vi "TraverseControl_High.vi"(0 "Mode":T2=enum."Read traverse position", 1 "Route Checking?":bool, 2 "Home":T1, 3 "Traverse Name":string, 7 "Model       Roll      Pitch       Yaw (deg)":dbl[](array[numeric]) format="%#.2f", 11 "Position input XYZ":dbl[](array[numeric])=[0.0, 0.0, 0.0] format="%.2f", 12 "Last Part of Move?":bool, 13 "Speed Factor":dbl=1.0 min=0.1 max=5.0 format="%.2f", 14 "Backlash Compensation?":bool=TRUE) -> (4 "Position Output XYZ":dbl[](array[numeric]) format="%.2f", 15 "Error String":string)   [LabVIEW 2014]
uses:
  Anemometry/Anemometry Sub Vis/Gen Trav/Trav_mode.ctl
  Anemometry/Anemometry Sub Vis/Controls/Home.ctl
  Anemometry/Anemometry Sub Vis/Globals/Trav_pos_global.vi
  Anemometry/Anemometry Sub Vis/Gen Trav/Route mapping/Route_mapping_global.vi
  Anemometry/Anemometry Sub Vis/Globals/Preference_global.vi
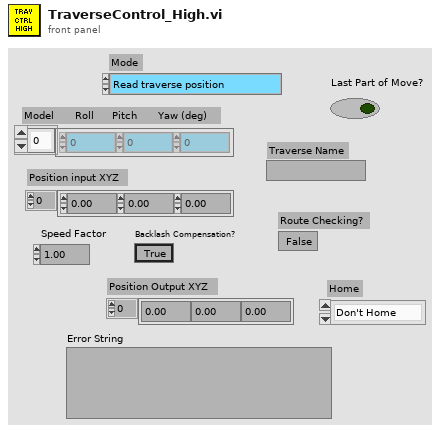
[diagram p1: front panel]
types:
  T1 = typedef "Home.ctl" = enum16{"Don't Home", "Home  +X", "Home  -X", "Home  +Y", "Home  -Y", "Home  +Z", "Home  -Z"}
  T2 = typedef "Trav_mode.ctl" = enum16{"Move traverse", "Read traverse position", "Teach Position"}
  T3 = typedef "Tunnel_Coordinates.ctl" = enum16{"Work in Tunnel Coordinates", "Work in Model Coordinates"}
  T4 = typedef "Box_size.ctl" = cluster{"Max":dbl, "Min":dbl}[]
  T5 = typedef "Exclude_cluster.ctl" = cluster{"Sizes":T4, "Name":string, "Exclude Type":T6}
  T6 = typedef "Exclusion_type.ctl" = enum16{"Exclude completely", "Allow only vertical moves"}
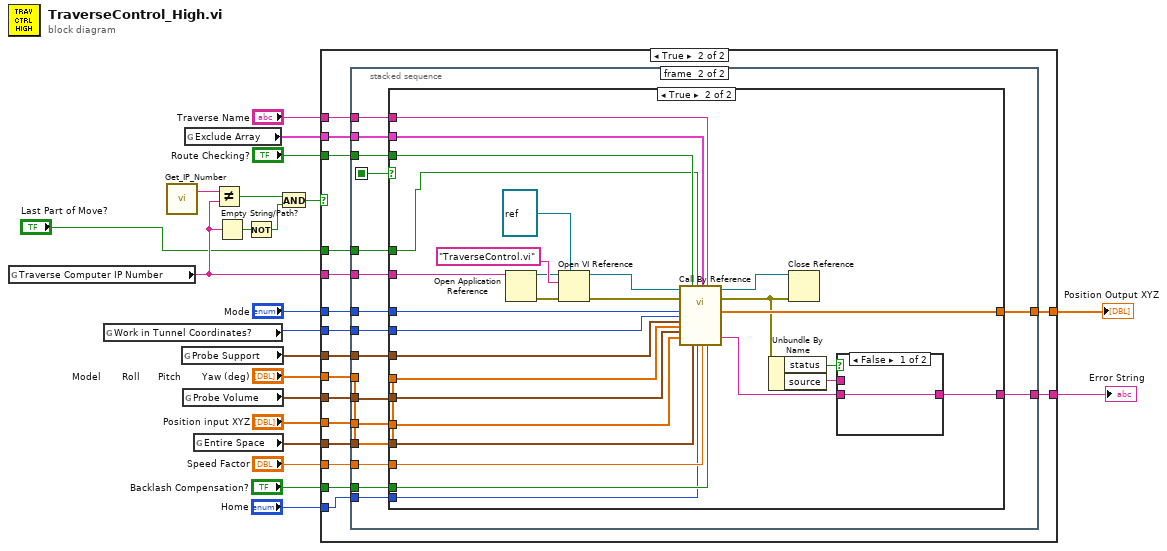
[diagram p0: block diagram]
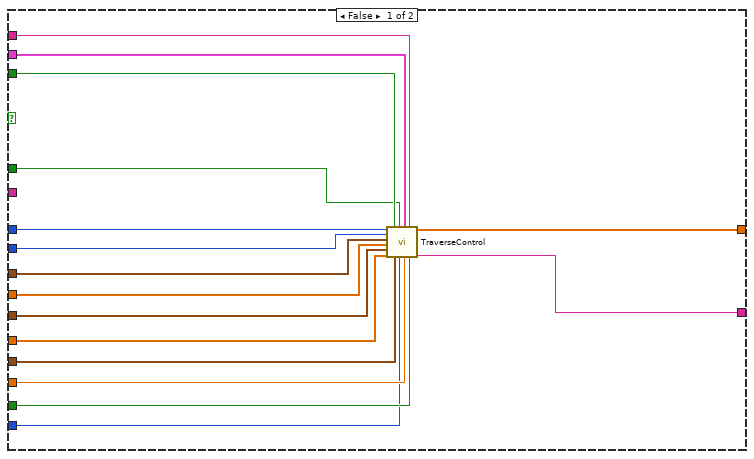
[diagram p2: hidden frame]
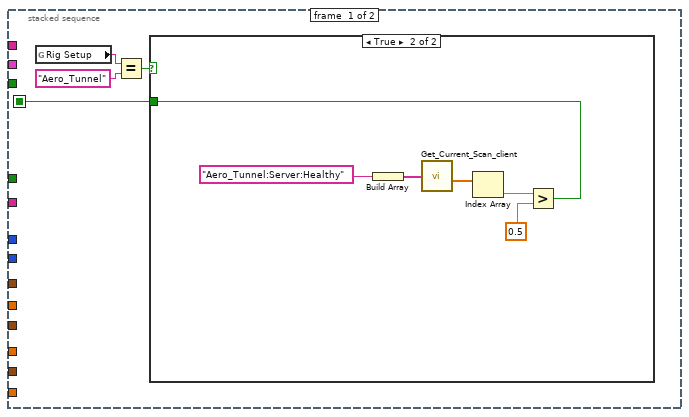
[diagram p3: hidden frame]
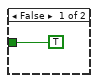
[diagram p4: hidden frame]
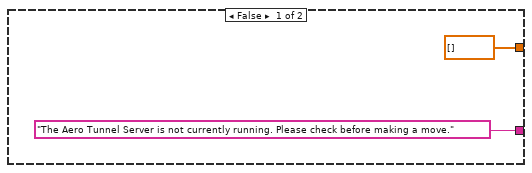
[diagram p5: hidden frame]
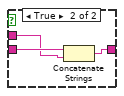
[diagram p6: hidden frame]
diagram:
  n1 = global read "Trav_pos_global.vi" "Traverse Computer IP Number"() -> (w10:string)
  n2 = global read "Trav_pos_global.vi" "Work in Tunnel Coordinates?"() -> (w4:T3)
  n3 = call "Get_IP_Number.vi"() -> ("IP Number"=w22:string)  [unwired: 1 out]
  n4 = global read "Route_mapping_global.vi" "Probe Support"() -> (w3:T4)
  n5 = global read "Route_mapping_global.vi" "Probe Volume"() -> (w5:T4)
  n6 = global read "Route_mapping_global.vi" "Exclude Array"() -> (w7:T5[])
  n7 = global read "Route_mapping_global.vi" "Entire Space"() -> (w6:T4)
  n8 = Not Equal?(x=w22, y=w10) -> (x != y?=w9:bool)
  n9 = Empty String/Path?(string/path=w10) -> (empty?=w12:bool)
  n10 = Not(x=w12) -> (.not. x?=w11:bool)
  n11 = And(x=w9, y=w11) -> (x .and. y?=w8:bool)
  n12 = case shown="True" w8 {
    tunnel: "Route Checking?" -> [w31 w55]
    tunnel: "Traverse Name" -> [w30 w54]
    tunnel: [w37 w53] -> w19
    tunnel: [w38 w45] -> w18
    tunnel: "Backlash Compensation?" -> [w34 w52]
    tunnel: "Speed Factor" -> [w33 w51]
    tunnel: "Position input XYZ" -> [w36 w50]
    tunnel: "Model       Roll      Pitch       Yaw (deg)" -> [w35 w49]
    tunnel: "Mode" -> [w32 w48]
    tunnel: w10 -> [_ w47]
    tunnel: w7 -> [w29 w46]
    tunnel: w6 -> [w28 w42]
    tunnel: w5 -> [w27 w43]
    tunnel: w4 -> [w26 w44]
    tunnel: w3 -> [w25 w41]
    tunnel: "Last Part of Move?" -> [w24 w40]
    tunnel: "Home" -> [w23 w39]
    frame False {
      n13 = call "TraverseControl.vi"("Mode"=w32, "Work in Tunnel Coordinates?"=w26, "Probe Support"=w25, "Model       Roll      Pitch       Yaw (deg)"=w35, "Probe Volume"=w27, "Position input XYZ"=w36, "Route Checking?"=w31, "Entire Space"=w28, "Last Part of Move?"=w24, "Home"=w23, "Exclude Array"=w29, "Speed Factor"=w33, "Traverse Name"=w30, "Backlash Compensation?"=w34) -> ("Position Output XYZ"=w37:dbl[], "Error String"=w38:string)  [unwired: 4 in]
    }
    frame True {
      n14 = stacked-sequence {
        seq-local: [w56 _] -> [_ w70]
        tunnel: w55 -> [_ w84]
        tunnel: w54 -> [_ w83]
        tunnel: [_ w82] -> w53
        tunnel: w52 -> [_ w81]
        tunnel: w51 -> [_ w80]
        tunnel: w50 -> [_ w79]
        tunnel: w49 -> [_ w78]
        tunnel: w48 -> [_ w77]
        tunnel: w47 -> [_ w76]
        tunnel: w46 -> [_ w75]
        tunnel: [_ w74] -> w45
        tunnel: w44 -> [_ w73]
        tunnel: w43 -> [_ w72]
        tunnel: w42 -> [_ w71]
        tunnel: w41 -> [_ w69]
        tunnel: w40 -> [_ w68]
        tunnel: w39 -> [_ w67]
        frame #0 {
          n15 = global read "Preference_global.vi" "Rig Setup"() -> (w59:string)
          n16 = Equal?(x=w59, y="Aero_Tunnel" ("Rig Setup")) -> (x = y?=w57:bool)
          n17 = case shown="True" w57 {
            tunnel: [TRUE w61] -> w56
            frame False {
            }
            frame True {
              n18 = Build Array("Aero_Tunnel:Server:Healthy") -> (w66:string[])
              n19 = call "Get_Current_Scan_client.vi"("ADAM Ch Names"=w66) -> ("Numerical Values"=w64:dbl[])  [unwired: 3 out]
              n20 = Index Array(array=w64) -> (element=w63:dbl)  [unwired: 1 in]
              n21 = Greater?(x=w63, y=0.5) -> (0:w61:bool)
            }
          }
        }
        frame #1 {
          n22 = case shown="True" w70 {
            tunnel: w84 -> [_ w111]
            tunnel: w83 -> [_ w110]
            tunnel: [dbl[] [] ("Position Output XYZ") w109] -> w82
            tunnel: w81 -> [_ w108]
            tunnel: w80 -> [_ w107]
            tunnel: w79 -> [_ w106]
            tunnel: w78 -> [_ w105]
            tunnel: w77 -> [_ w104]
            tunnel: w76 -> [_ w101]
            tunnel: w75 -> [_ w98]
            tunnel: ["The Aero Tunnel Server is not currently running. Please check before making a move." ("Error String") w95] -> w74
            tunnel: w73 -> [_ w92]
            tunnel: w72 -> [_ w91]
            tunnel: w71 -> [_ w90]
            tunnel: w69 -> [_ w89]
            tunnel: w68 -> [_ w88]
            tunnel: w67 -> [_ w87]
            frame False {
            }
            frame True {
              n23 = Open Application Reference(11:w101) -> (0:w99:errorcluster, 3:w100:refnum<vi>)  [unwired: 2 in, 1 out]
              n24 = Open VI Reference(type specifier VI Refnum (for type only)=refnum<vi> refnum ("Scout Server"), application reference (local)=w100, vi path="TraverseControl.vi", error in (no error)=w99) -> (vi reference=w112:refnum<vi>, error out=w103:errorcluster)  [unwired: 2 out]
              n25 = call-by-ref "?"(reference=w112, error in=w103, "Mode"=w104, "Work in Tunnel Coordinates?"=w92, "Probe Support"=w89, "Model       Roll      Pitch       Yaw (deg)"=w105, "Probe Volume"=w91, "Position input XYZ"=w106, "Route Checking?"=w111, "Entire Space"=w90, "Last Part of Move?"=w88, "Home"=w87, "Exclude Array"=w98, "Speed Factor"=w107, "Traverse Name"=w110, "Backlash Compensation?"=w108) -> (reference out=w102:refnum<vi>, error out=w97:errorcluster, "Position Output XYZ"=w109:dbl[], "Error String"=w94:string)  [unwired: 4 in]
              n26 = Unbundle By Name(w97) -> ("status"=w96:bool, "source"=w93:string)
              n27 = Close Reference(reference=w102, error in (no error)=w97) -> ()  [unwired: 1 out]
              n28 = case shown="False" w96 {
                tunnel: [w115 w118] -> w95
                tunnel: w94 -> [w115 w117]
                tunnel: w93 -> [_ w116]
                frame False {
                }
                frame True {
                  n29 = Concatenate Strings(w117, w116) -> (w118:string)
                }
              }
            }
          }
        }
      }
    }
  }
  "Error String" <- w18
  "Position Output XYZ" <- w19
